vi "ReconnectIfError.vi"(6 "TryReconnect":bool, 7 "ConnectionTimeout":i32, 8 "error in (no error)":errorcluster, 9 "Port":u16, 10 "IP-Address":string, 11 "TCP Network Connection in":refnum<k5>) -> (0 "error out":errorcluster, 2 "TryAgain(Managed to Reconnect, and TryReconnect is True)":bool, 3 "TCP Network Connection out":refnum<k5>)   [LabVIEW 2020, in "VdTcpIP.lvclass"]
uses:
  VdTcpIP.lvclass
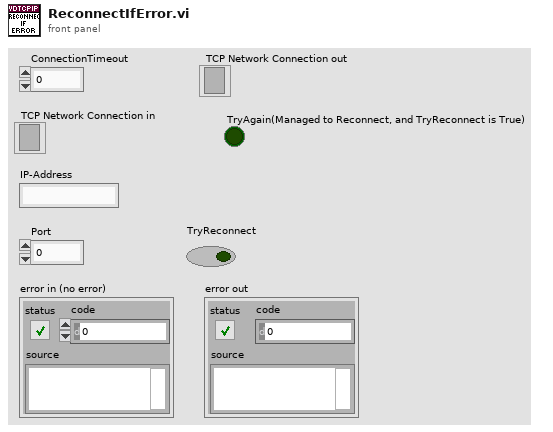
[diagram p1: front panel]
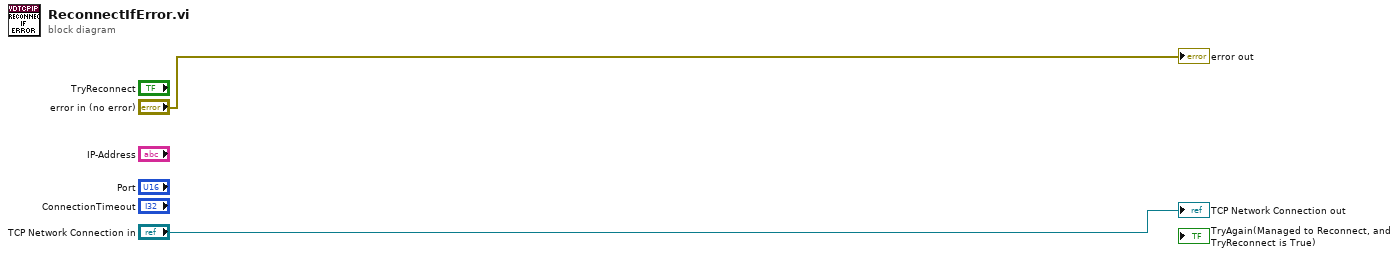
[diagram p0: block diagram]
diagram:
  "error out" <- "error in (no error)"
  "TCP Network Connection out" <- "TCP Network Connection in"
